vi "OSC Sender.vi"(8 "Mode":bool, 9 "Value":dbl format="%#_13g", 10 "Label":string, 11 "State":enum16{"Init", "Send", "Mode"}(ring)=enum."Send") -> ()   [LabVIEW 2016]
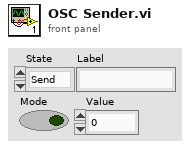
[diagram p1: front panel]
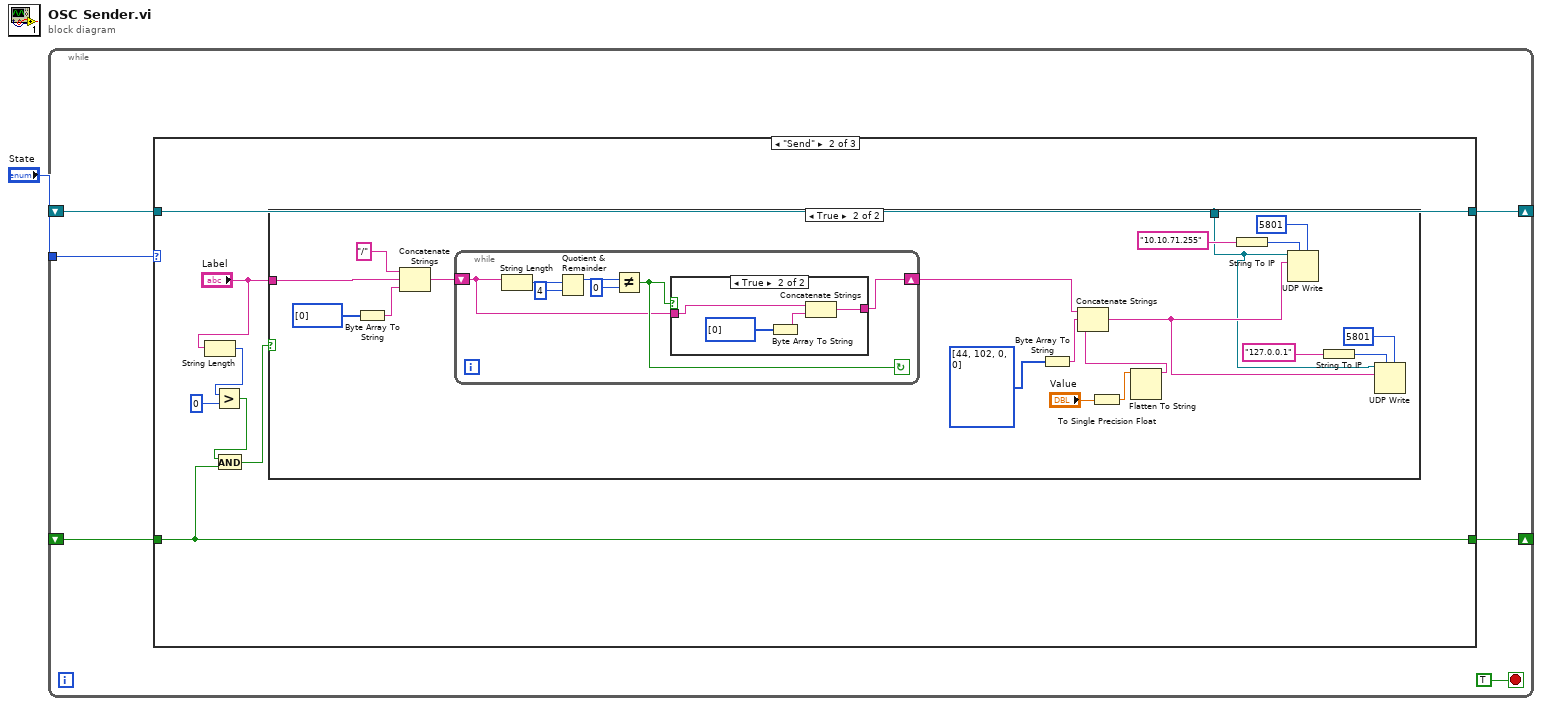
[diagram p0: block diagram]
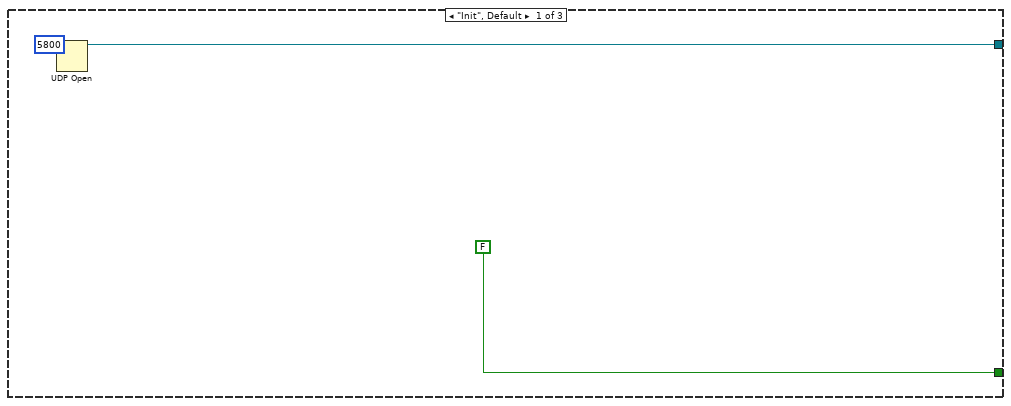
[diagram p2: hidden frame]
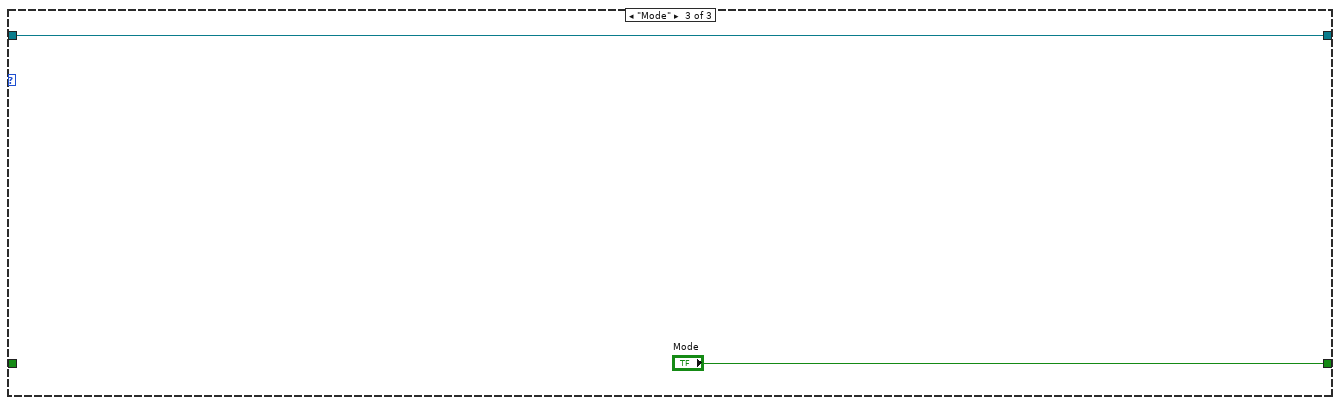
[diagram p5: hidden frame]
diagram:
  n1 = while {
    tunnel: "State" -> [w7]
    shift-right: [w6] -> _
    shift-left: _ -> [w3]
    shift-right: [w5] -> _
    shift-left: _ -> [w4]
    stop <- TRUE stop-if-true
    n2 = case shown="\"Send\"" w7 {
      tunnel: [w9 w17 w49] -> w6
      tunnel: [FALSE ("Boolean") w16 "Mode"] -> w5
      tunnel: w4 -> [_ w16 _]
      tunnel: w3 -> [_ w17 w49]
      frame "Init", Default {
        n3 = UDP Open(11:u16 5800 ("port")) -> (port=w9:refnum<k16>)  [unwired: 4 in, 2 out]
      }
      frame "Send" {
        n4 = String Length(string="Label") -> (length=w14:i32)
        n5 = Greater?(x=w14, y=0) -> (0:w12:bool)
        n6 = And(x=w12, y=w16) -> (x .and. y?=w11:bool)
        n7 = case shown="True" w11 {
          tunnel: "Label" -> [_ w35]
          tunnel: w17 -> [_ w18]
          frame False {
          }
          frame True {
            n8 = Byte Array To String(unsigned byte array=u8[] [0]) -> (string=w33:string)
            n9 = Concatenate Strings("/" ("string"), w35, w33) -> (w31:string)
            n10 = while {
              shift-right: [w37] -> w29
              shift-left: w31 -> [w38]
              stop <- w39 continue-if-true
              n11 = String Length(string=w38) -> (length=w43:i32)
              n12 = Quotient & Remainder(x=w43, y=4) -> (x-y*floor(x/y)=w41:i32)  [unwired: 1 out]
              n13 = Not Equal?(x=w41, y=0) -> (x != y?=w39:bool)
              n14 = case shown="True" w39 {
                tunnel: [w44 w45] -> w37
                tunnel: w38 -> [w44 w47]
                frame False {
                }
                frame True {
                  n15 = Byte Array To String(unsigned byte array=u8[] [0]) -> (string=w46:string)
                  n16 = Concatenate Strings(w47, w46) -> (w45:string)
                }
              }
            }
            n17 = Byte Array To String(unsigned byte array=u8[] [44, 102, 0, 0]) -> (string=w28:string)
            n18 = To Single Precision Float(number="Value") -> (single precision float=w27:sgl)
            n19 = Flatten To String(anything=w27) -> (data string=w26:string)  [unwired: 3 in, 2 out]
            n20 = Concatenate Strings(w29, w28, w26) -> (w19:string)
            n21 = String To IP(1:"10.10.71.255" ("name")) -> (0:w24:u32)
            n22 = UDP Write(address=w24, port or service name=u16 5801, connection ID=w18, data in=w19) -> ()  [unwired: 2 in, 2 out]
            n23 = String To IP(1:"127.0.0.1" ("name")) -> (0:w21:u32)
            n24 = UDP Write(address=w21, port or service name=u16 5801, connection ID=w18, data in=w19) -> ()  [unwired: 2 in, 2 out]
          }
        }
      }
      frame "Mode" {
      }
    }
  }
